vi "RepositionItemsWithinCaseStructure.vi"(8 "error in (no error)":errorcluster, 9 "Items inside case structure":refnum<vi>[](array[refnum]), 10 "New case structure ref":refnum<vi>, 11 "VI ref in":refnum<vi>) -> (0 "error out":errorcluster, 2 "New case structure ref (dup)":refnum<vi>, 3 "VI ref out (dup)":refnum<vi>)   [LabVIEW 2017, in "ErrorStructureDrawer.lvlib"]
doc: "Resizes the new case structure and positions its contents"
uses:
  ErrorStructureDrawer.lvlib
  <vilib>/Utility/miscctls.llb/LVDeltaXY32Cluster.ctl
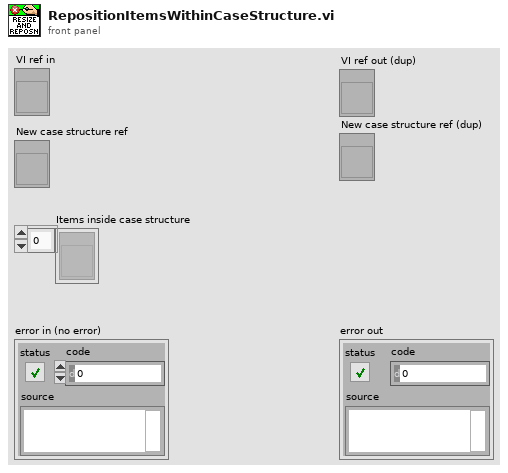
[diagram p1: front panel]
types:
  T1 = typedef "LVDeltaXY32Cluster.ctl" = cluster{"X":i32, "Y":i32}
  T2 = typedef "LVBoundsTypeDef.ctl" = cluster{"Width":u32, "Height":u32}
  T3 = typedef "LVPositionTypeDef.ctl" = cluster{"Left":i32, "Top":i32}
  T4 = typedef "LVRectTypeDef.ctl" = cluster{"Left":i16, "Top":i16, "Right":i16, "Bottom":i16}
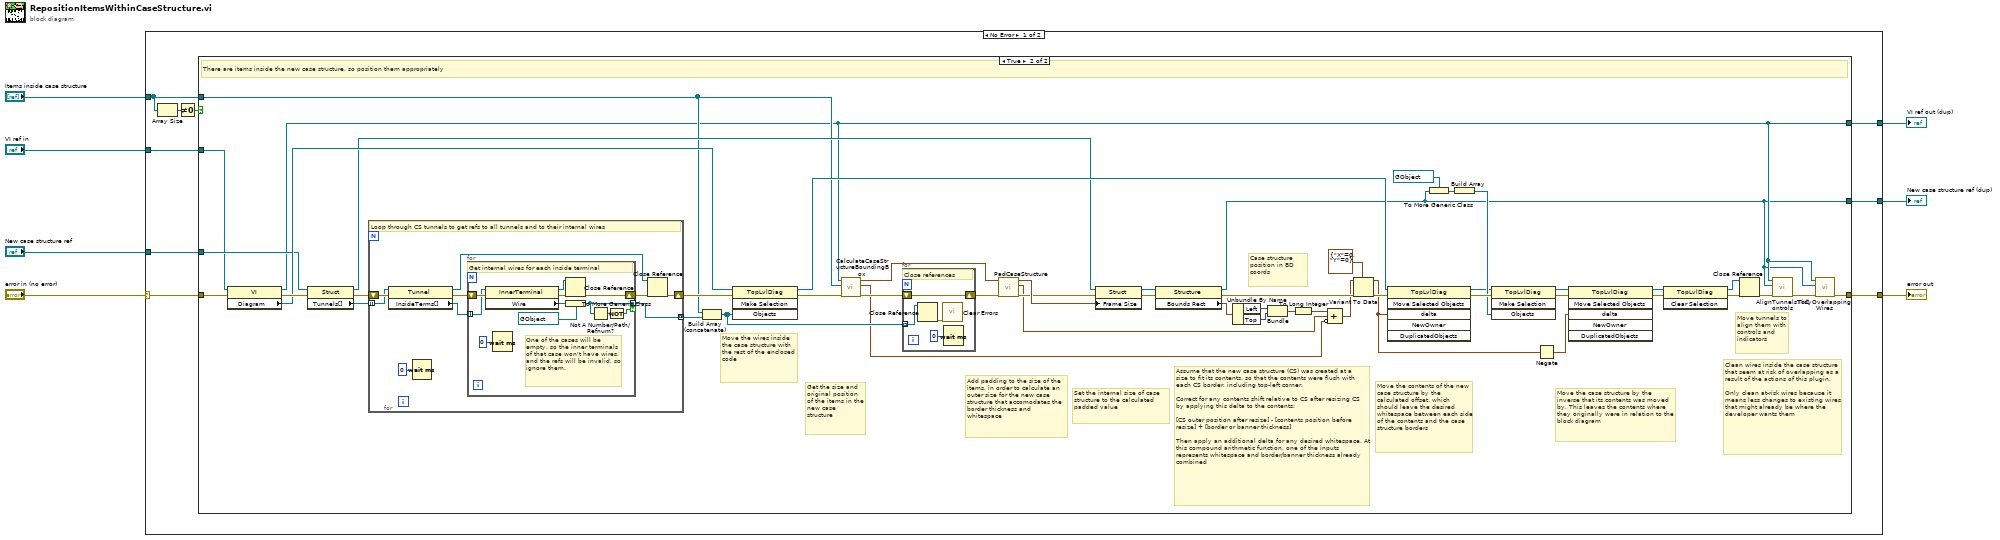
[diagram p0: block diagram]
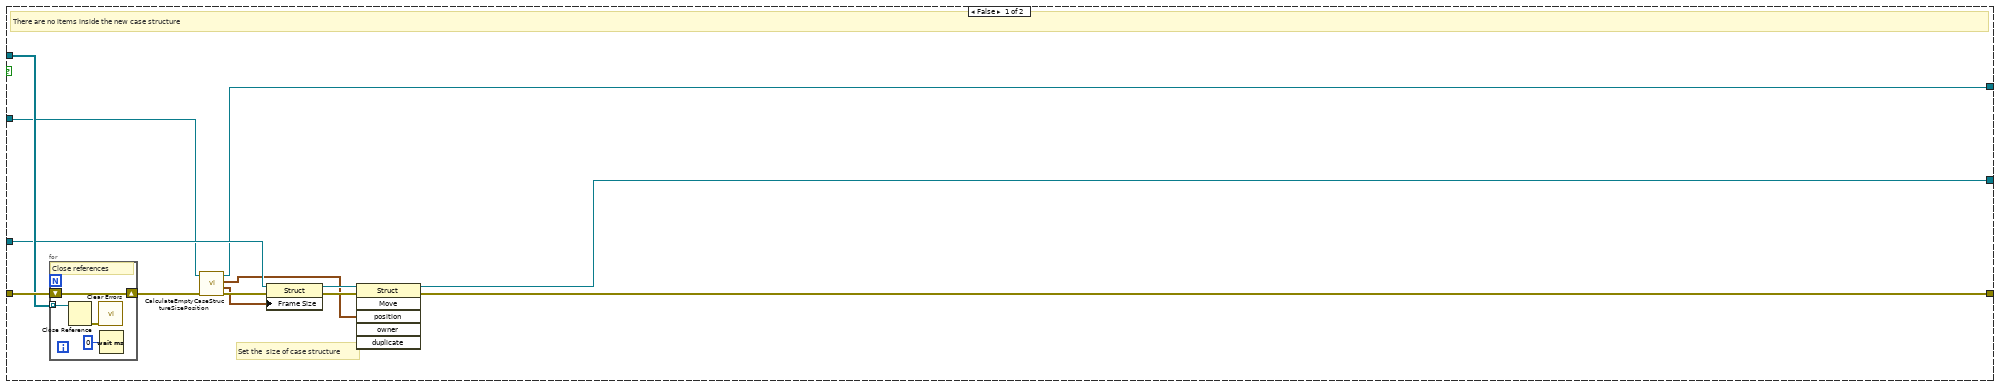
[diagram p2: hidden frame]
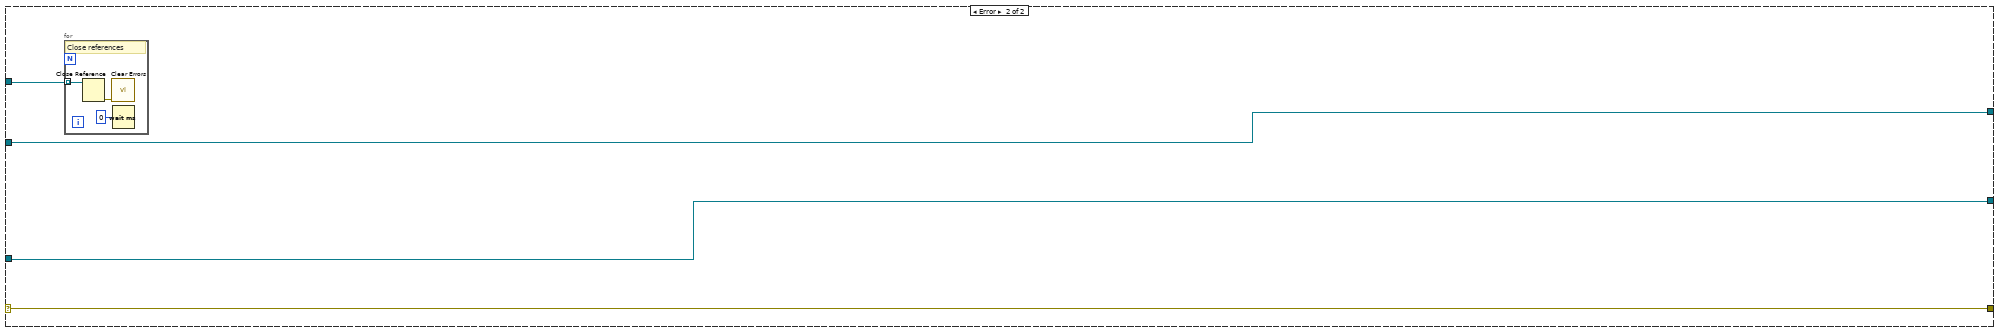
[diagram p3: hidden frame]
diagram:
  n1 = case shown="No Error" "error in (no error)" {
    selector: "error in (no error)" -> [w11 w111]
    tunnel: "New case structure ref" -> [w16 w110]
    tunnel: [w15 w111] -> w6
    tunnel: "Items inside case structure" -> [w10 w108]
    tunnel: "VI ref in" -> [w14 w109]
    tunnel: [w13 w109] -> w3
    tunnel: [w12 w110] -> w2
    frame No Error {
      n2 = Array Size(array=w10) -> (size(s)=w9:i32)
      n3 = Not Equal To 0?(x=w9) -> (x != 0?=w8:bool)
      n4 = case shown="True" w8 {
        tunnel: w16 -> [w22 w60]
        tunnel: [w26 w36] -> w15
        tunnel: w10 -> [w27 w39]
        tunnel: w14 -> [w20 w51]
        tunnel: [w19 w35] -> w13
        tunnel: [w17 w34] -> w12
        tunnel: w11 -> [w28 w46]
        frame False {
          # "Set the  size of case structure"
          # "There are no items inside the new case structure"
          n5 = for {
            tunnel: w27 -> [w31] mode=indexing
            shift-right: [w32] -> w21
            shift-left: w28 -> [w32]
            # "Close references"
            n6 = Close Reference(reference=w31) -> (error out=w33:errorcluster)  [unwired: 1 in]
            n7 = call <vilib>:"Clear Errors.vi"("error in (no error)"=w33) -> ()  [unwired: 5 in, 2 out]
            n8 = Wait (ms)(milliseconds to wait=u32 0) -> ()  [unwired: 1 out]
          }
          n9 = call "CalculateEmptyCaseStructureSizePosition.vi"("error in (no error)"=w21, "VI ref in"=w20) -> ("error out"=w25:errorcluster, "Case structure frame size"=w24:T2, "Case structure position"=w18:T3, "VI ref (dup)"=w19:refnum<vi>)  [unwired: 6 in]
          n10 = property class="Struct"(reference=w22, error in=w25, "Frame Size"=w24) -> (reference out=w23:refnum<vi>, error out=w29:errorcluster)
          n11 = invoke class="Struct" method="Move"(reference=w23, error in=w29, "position"=w18) -> (reference out=w17:refnum<vi>, error out=w26:errorcluster)  [unwired: 3 in, 4 out]
        }
        frame True {
          # "Clean wires inside the case structure that seem at risk of overlapping as a result of the actions of this plugin.\n\nOnly clean at-risk wires because it means less changes to existing wires that might already be where the developer wants them"
          # "Move tunnels to align them with controls and indicators"
          # "Move the wires inside the case structure with the rest of the enclosed code"
          # "Move the case structure by the inverse that its contents was moved by. This leaves the contents where they originally were in relation to the block diagram"
          # "Assume that the new case structure (CS) was created at a size to fit its contents, so that the contents were flush with each CS border, including top-left corner.\n\nCorrect for any contents shift relative to CS after resizing CS by applying this delta to the contents:\n\n[CS outer position after resize] - [contents position before resize] + [border or banner thickness]\n\nThen apply an additional delta for any desired whitespace. At this compound arithmetic function, one of the inputs represents whitespace and border/banner thickness already combined"
          # "Case structure position in BD coords"
          # "Move the contents of the new case structure by the calculated offset, which should leave the desired whitespace between each side of the contents and the case structure borders"
          # "Set the internal size of case structure to the calculated padded value"
          # "Add padding to the size of the items, in order to calculate an outer size for the new case structure that accomodates the border thickness and whitespace"
          # "Get the size and original position of the items in the new case structure"
          # "There are items inside the new case structure, so position them appropriately"
          n12 = property class="VI"(reference=w51, error in=w46) -> (reference out=w35:refnum<vi>, error out=w82:errorcluster, "Diagram"=w67:refnum<vi>)
          n13 = property class="Struct"(reference=w60, error in=w82) -> (reference out=w59:refnum<vi>, error out=w50:errorcluster, "Tunnels[]"=w58:refnum<vi>[])
          n14 = for {
            tunnel: w58 -> [w91] mode=indexing
            tunnel: [w92] -> w57 mode=concatenating
            shift-right: [w89] -> w49
            shift-left: w50 -> [w94]
            # "Loop through CS tunnels to get refs to all tunnels and to their internal wires"
            n15 = property class="Tunnel"(reference=w91, error in=w94) -> (reference out=w88:refnum<vi>, error out=w96:errorcluster, "InsideTerms[]"=w95:refnum<vi>[])
            n16 = Wait (ms)(milliseconds to wait=u32 0) -> ()  [unwired: 1 out]
            n17 = for {
              tunnel: w95 -> [w106] mode=indexing
              tunnel: [w103] -> w92 mode=indexing if=w101
              shift-right: [w99] -> w90
              shift-left: w96 -> [w107]
              # "One of the cases will be empty, so the inner terminals of that case won't have wires, and the refs will be invalid, so ignore them."
              # "Get internal wires for each inside terminal"
              n18 = property class="InnerTerminal"(reference=w106, error in=w107) -> (reference out=w98:refnum<vi>, error out=w100:errorcluster, "Wire"=w104:refnum<vi>)
              n19 = Wait (ms)(milliseconds to wait=u32 0) -> ()  [unwired: 1 out]
              n20 = Close Reference(reference=w98, error in (no error)=w100) -> (error out=w99:errorcluster)
              n21 = To More Generic Class(target class=refnum<vi> refnum, reference=w104) -> (generic class reference=w103:refnum<vi>)
              n22 = Not A Number/Path/Refnum?(number/path/refnum=w103) -> (NaN/Path/Refnum?=w102:bool)
              n23 = Not(x=w102) -> (.not. x?=w101:bool)
            }
            n24 = Close Reference(reference=w88, error in (no error)=w90) -> (error out=w89:errorcluster)
          }
          n25 = Build Array (concatenate)(w39, w57) -> (w47:refnum<vi>[])
          n26 = invoke class="TopLvlDiag" method="Make Selection"(reference=w67, error in=w49, "Objects"=w47) -> (reference out=w64:refnum<vi>, error out=w43:errorcluster)  [unwired: 1 in, 2 out]
          n27 = call "CalculateCaseStructureBoundingBox.vi"("Error In"=w43, "Items to enclose in case structure"=w39, "VI reference"=w35) -> ("Error Out"=w42:errorcluster, "Current bounding box position"=w40:cluster{"Left":i32, "Top":i32}, "Size of bounding box for items"=w41:T2)  [unwired: 6 in]
          n28 = for {
            tunnel: w47 -> [w85] mode=indexing
            shift-right: [w86] -> w48
            shift-left: w42 -> [w86]
            # "Close references"
            n29 = Close Reference(reference=w85) -> (error out=w87:errorcluster)  [unwired: 1 in]
            n30 = call <vilib>:"Clear Errors.vi"("error in (no error)"=w87) -> ()  [unwired: 5 in, 2 out]
            n31 = Wait (ms)(milliseconds to wait=u32 0) -> ()  [unwired: 1 out]
          }
          n32 = call "PadCaseStructure.vi"("error in (no error)"=w48, "Bounding box for items in"=w41) -> ("error out"=w74:errorcluster, "Offset for items from outer top left corner"=w72:cluster{"Horizontal":i32, "Vertical":i32}, "Padded bounding box for items"=w76:T2)  [unwired: 7 in]
          n33 = property class="Struct"(reference=w59, error in=w74, "Frame Size"=w76) -> (reference out=w68:refnum<vi>, error out=w75:errorcluster)
          n34 = property class="Structure"(reference=w68, error in=w75) -> (reference out=w34:refnum<vi>, error out=w81:errorcluster, "Bounds Rect"=w77:T4)
          n35 = Unbundle By Name(w77) -> ("Left"=w78:i16, "Top"=w79:i16)
          n36 = Bundle("Left"=w78, "Top"=w79) -> (w80:cluster{"Left":i16, "Top":i16})  [unwired: 1 in]
          n37 = To Long Integer(number=w80) -> (32bit integer=w73:cluster{"Left":i32, "Top":i32})
          n38 = Compound Arithmetic op=ADD(w73, w72, invert w40) -> (w71:cluster{i32, i32})
          n39 = Variant To Data(error in=w81, type=T1 {"X"=0, "Y"=0} ("X/Y Delta"), Variant=w71) -> (data=w44:T1, error out=w70:errorcluster)
          n40 = invoke class="TopLvlDiag" method="Move Selected Objects"(reference=w64, error in=w70, "delta"=w44) -> (reference out=w45:refnum<vi>, error out=w83:errorcluster)  [unwired: 3 in, 4 out]
          n41 = To More Generic Class(target class=refnum<vi> refnum, reference=w34) -> (generic class reference=w52:refnum<vi>)
          n42 = Build Array(w52) -> (w63:refnum<vi>[])
          n43 = invoke class="TopLvlDiag" method="Make Selection"(reference=w45, error in=w83, "Objects"=w63) -> (reference out=w66:refnum<vi>, error out=w65:errorcluster)  [unwired: 1 in, 2 out]
          n44 = Negate(x=w44) -> (-x=w62:T1)
          n45 = invoke class="TopLvlDiag" method="Move Selected Objects"(reference=w66, error in=w65, "delta"=w62) -> (reference out=w55:refnum<vi>, error out=w61:errorcluster)  [unwired: 3 in, 4 out]
          n46 = invoke class="TopLvlDiag" method="Clear Selection"(reference=w55, error in=w61) -> (reference out=w54:refnum<vi>, error out=w56:errorcluster)  [unwired: 1 in, 1 out]
          n47 = Close Reference(reference=w54, error in (no error)=w56) -> (error out=w38:errorcluster)
          n48 = call "AlignTunnelsToControls.vi"("Error In"=w38, "New case structure ref"=w34, "VI ref in"=w35) -> ("Error Out"=w37:errorcluster)  [unwired: 8 in]
          n49 = call "TidyOverlappingWires.vi"("Error In"=w37, "New case structure ref"=w34, "VI ref in"=w35) -> ("Error Out"=w36:errorcluster)  [unwired: 8 in]
        }
      }
    }
    frame Error {
      n50 = for {
        tunnel: w108 -> [w113] mode=indexing
        # "Close references"
        n51 = Close Reference(reference=w113) -> (error out=w114:errorcluster)  [unwired: 1 in]
        n52 = call <vilib>:"Clear Errors.vi"("error in (no error)"=w114) -> ()  [unwired: 5 in, 2 out]
        n53 = Wait (ms)(milliseconds to wait=u32 0) -> ()  [unwired: 1 out]
      }
    }
  }
  "error out" <- w6
  "VI ref out (dup)" <- w3
  "New case structure ref (dup)" <- w2
